vi "Convert CAN Frame to RAW Frame.vi"(4 "CAN frame":T1={"timestamp"=timestamp(0 s since 1904-01-01), "payload"=[0, 0, 0, 0, 0, 0, 0, 0], "identifier"=0, "type"=0, "extended?"=FALSE, "echo?"=FALSE} {"payload" format="%x"; "timestamp" format="%<%.7X\n%x>T"; "type" items=["CAN Data"=0, "CAN Remote"=1, "CAN Bus Error"=2, "CAN 2.0 Data"=8, "CAN FD Data"=16, "CAN FD+BRS Data"=24, "J1939 Data"=192, "Delay"=224, "Log Trigger"=225, "Start Trigger"=226]; "identifier" format="%x"}) -> (1 "RAW Data":u8[](array[numeric]) format="%.0x")   [LabVIEW 2015, in "J1939 Addon Engine.lvlib"]
uses:
  J1939 Addon Engine.lvlib
  <vilib>/xnet/xnet.llb/XNET Frame CAN.ctl
  <vilib>/xnet/xnet.llb/XNET Frame Type CAN.ctl
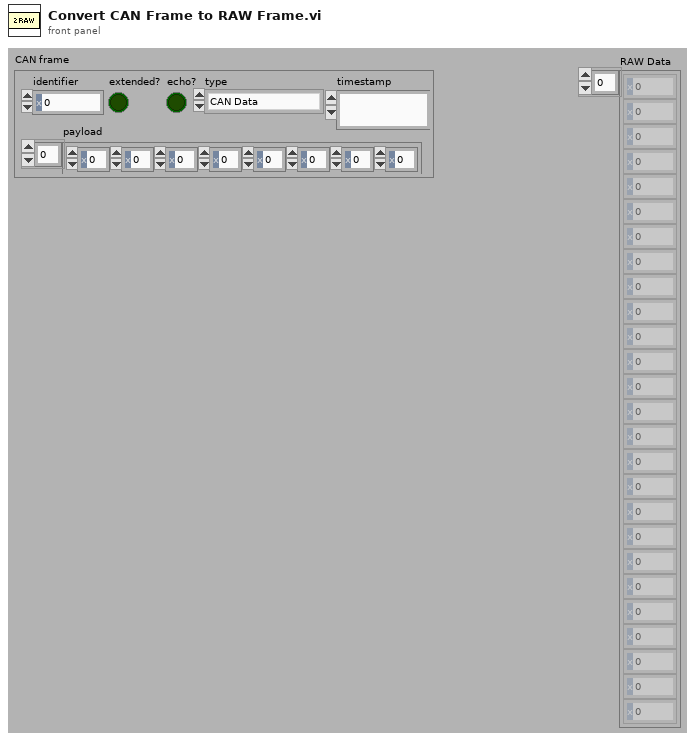
[diagram p1: front panel]
types:
  T1 = typedef "XNET Frame CAN.ctl" = cluster{"timestamp":timestamp, "payload":u8[], "identifier":u32, "type":T2, "extended?":bool, "echo?":bool}
  T2 = typedef "XNET Frame Type CAN.ctl" = u8
  T3 = enum16{"big-endian, network order", "native, host order", "little-endian"}
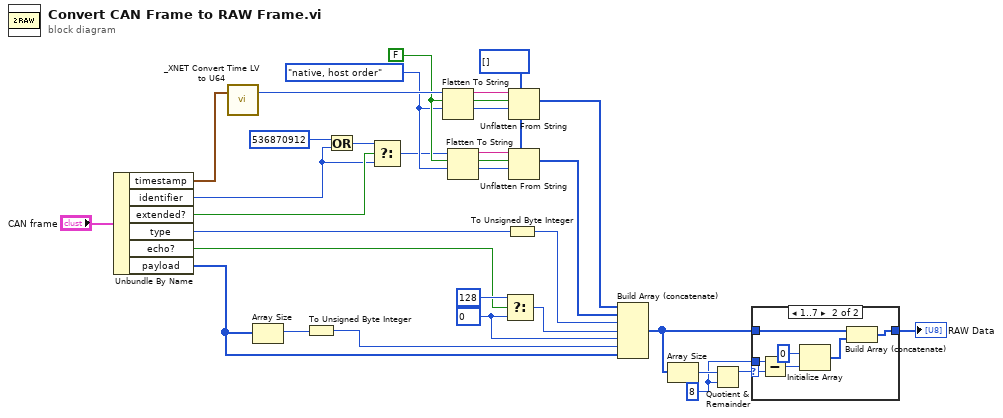
[diagram p0: block diagram]
diagram:
  w7 = 8 ("y")
  w12 = u8 0
  w9 = u8[] [] ("subarray")
  w24 = FALSE ("prepend array or string size? (T)")
  w23 = T3."native, host order" ("byte order (0:big-endian, network order)")
  n1 = Unbundle By Name("CAN frame") -> ("timestamp"=w29:timestamp, "identifier"=w18:u32, "extended?"=w20:bool, "type"=w10:T2, "echo?"=w15:bool, "payload"=w13:u8[])
  n2 = call <vilib>:"_XNET Convert Time LV to U64.vi"("Time LV"=w29) -> ("Time U64"=w28:u64)  [unwired: 2 in]
  n3 = Array Size(array=w13) -> (size(s)=w11:i32)
  n4 = To Unsigned Byte Integer(number=w11) -> (unsigned 8bit integer=w2:u8)
  n5 = Or(x=u32 536870912, y=w18) -> (x .or. y?=w19:u32)
  n6 = Select(t=w19, s=w20, f=w18) -> (s? t:f=w17:u32)
  n7 = Flatten To String(anything=w28, prepend array or string size? (T)=w24, byte order (0:big-endian, network order)=w23) -> (data string=w27:string)  [unwired: 1 in, 2 out]
  n8 = Flatten To String(anything=w17, prepend array or string size? (T)=w24, byte order (0:big-endian, network order)=w23) -> (data string=w25:string)  [unwired: 1 in, 2 out]
  n9 = Select(t=u8 128, s=w15, f=w12) -> (s? t:f=w14:u8)
  n10 = To Unsigned Byte Integer(number=w10) -> (unsigned 8bit integer=w1:T2)
  n11 = Unflatten From String(type=w9, binary string=w27, data includes array or string size? (T)=w24, byte order (0:big-endian, network order)=w23) -> (value=w26:u8[])  [unwired: 1 in, 2 out]
  n12 = Unflatten From String(type=w9, binary string=w25, data includes array or string size? (T)=w24, byte order (0:big-endian, network order)=w23) -> (value=w22:u8[])  [unwired: 1 in, 2 out]
  n13 = Build Array (concatenate)(w26, w22, w1, w14, w12, w2, w13) -> (w5:T2[])
  n14 = Array Size(array=w5) -> (size(s)=w8:i32)
  n15 = Quotient & Remainder(x=w8, y=w7) -> (x-y*floor(x/y)=w6:i32)  [unwired: 1 out]
  n16 = case shown="1..7" w6 {
    selector: w6 -> [_ w31]
    tunnel: w7 -> [_ w37]
    tunnel: w5 -> [w30 w33]
    tunnel: [w30 w32] -> w4
    frame 0, Default {
    }
    frame 1..7 {
      n17 = Subtract(x=w37, y=w31) -> (x-y=w36:i32)
      n18 = Initialize Array(u8 0 ("Numeric"), w36) -> (w34:u8[])
      n19 = Build Array (concatenate)(w33, w34) -> (w32:T2[])
    }
  }
  "RAW Data" <- w4
